vi "create_measure_log_entry.vi"(0 "Messlogbuch-Pfad":path, 1 "Probe":string, 2 "Polarisation [°]":dbl, 3 "Messart":string, 4 "ROI":i32[](array[numeric]), 5 "error in":errorcluster, 6 "Messungen/Messschritt":i32, 7 "Maximalleistung (iK) [mW]":dbl, 8 "Tip-Spannung [V]":dbl, 9 "Suppressor-Spannung [V]":dbl, 10 "Zeit/Messschritt [ms]":i32, 11 "MCP-Spannung [V]":dbl, 12 "Zeit/Messung [ms]":i32, 13 "Phosphorschirm-Spannung [V]":dbl, 15 "xyz [mm]":dbl[](array[numeric])) -> (14 "Messung Nr.":i32, 19 "error out":errorcluster)   [LabVIEW 2009]
panel:
  out "Gestartet":timestamp
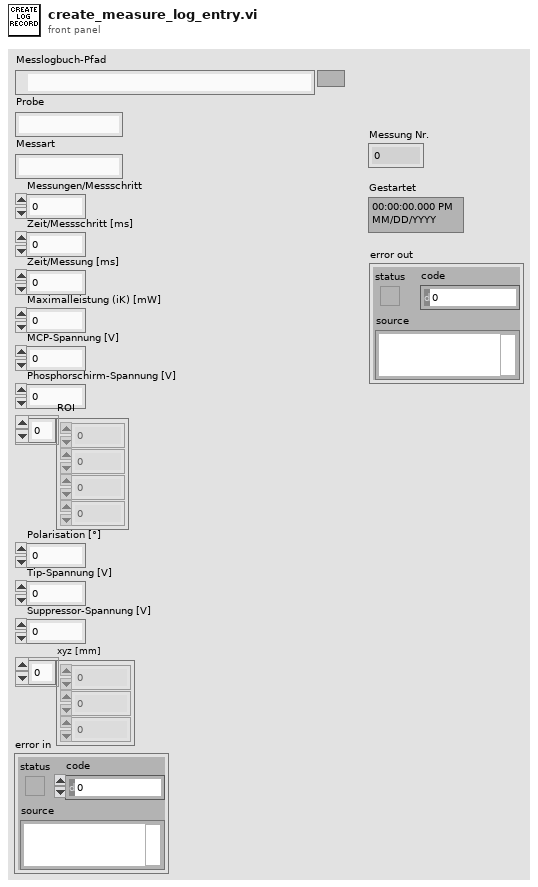
[diagram p1: front panel]
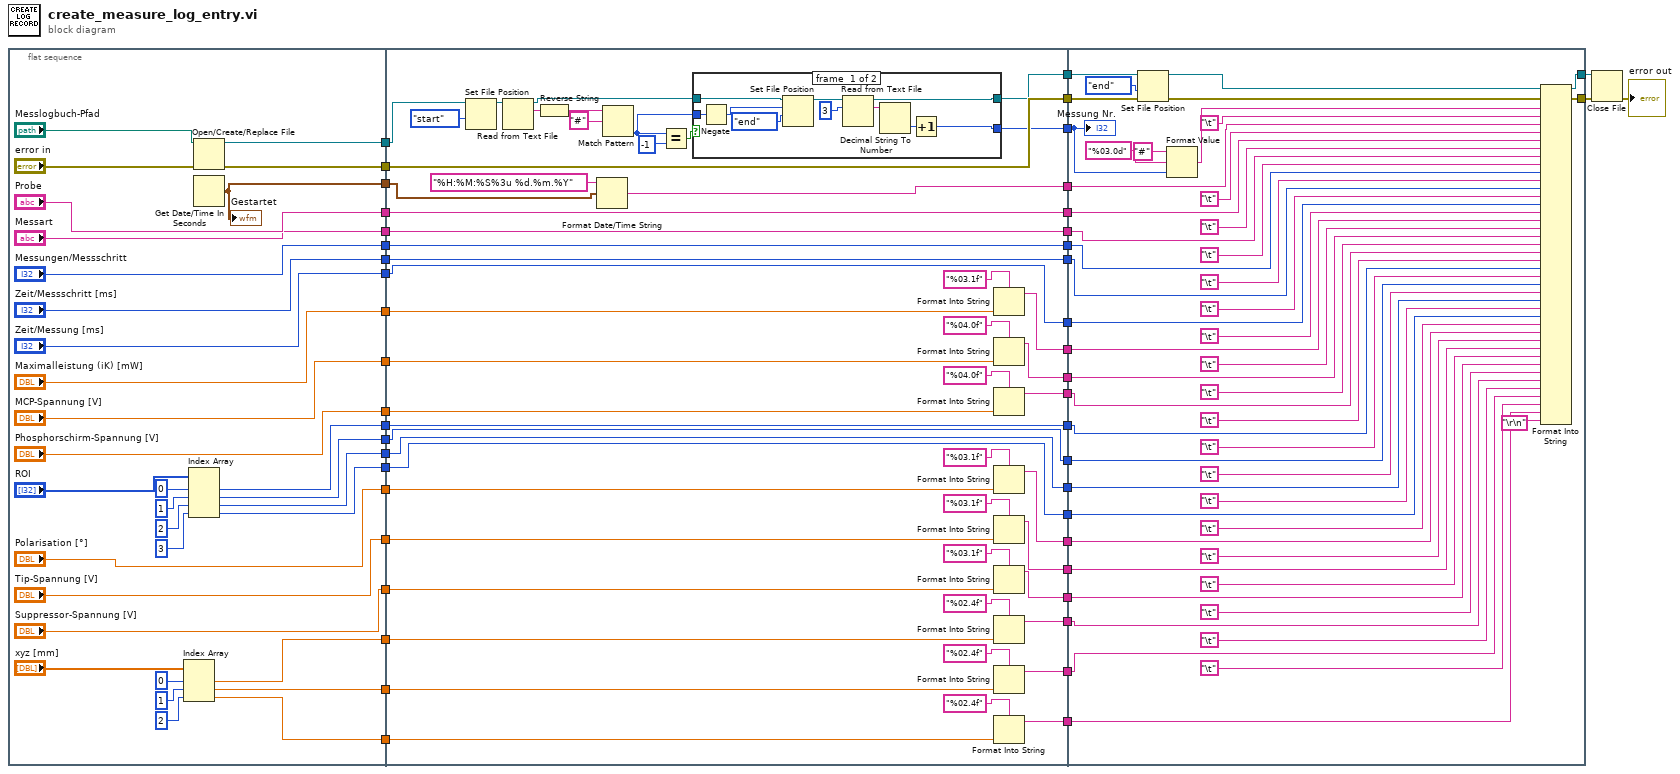
[diagram p0: block diagram]
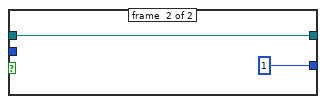
[diagram p2: hidden frame]
diagram:
  n1 = flat-sequence {
    tunnel: ["Probe"] -> w44
    tunnel: ["Messart"] -> w42
    tunnel: ["Messungen/Messschritt"] -> w40
    tunnel: ["Zeit/Messschritt [ms]"] -> w38
    tunnel: ["Zeit/Messung [ms]"] -> w36
    tunnel: ["Maximalleistung (iK) [mW]"] -> w34
    tunnel: ["MCP-Spannung [V]"] -> w32
    tunnel: ["Phosphorschirm-Spannung [V]"] -> w30
    tunnel: [w60] -> w28
    tunnel: [w59] -> w26
    tunnel: [w58] -> w24
    tunnel: [w57] -> w22
    tunnel: [w70] -> w20
    tunnel: [w68] -> w19
    tunnel: [w67] -> w18
    tunnel: ["Polarisation [°]"] -> w12
    tunnel: ["Tip-Spannung [V]"] -> w10
    tunnel: ["Suppressor-Spannung [V]"] -> w8
    tunnel: [w49] -> w6
    tunnel: [w48] -> w4
    tunnel: [w47] -> w2
    tunnel: w44 -> [w130]
    tunnel: [w130] -> w43
    tunnel: w42 -> [w129]
    tunnel: [w129] -> w41
    tunnel: w40 -> [w128]
    tunnel: [w128] -> w39
    tunnel: w38 -> [w127]
    tunnel: [w127] -> w37
    tunnel: w36 -> [w126]
    tunnel: [w126] -> w35
    tunnel: w34 -> [w107]
    tunnel: [w106] -> w33
    tunnel: w32 -> [w101]
    tunnel: [w100] -> w31
    tunnel: w30 -> [w103]
    tunnel: [w102] -> w29
    tunnel: w28 -> [w125]
    tunnel: [w125] -> w27
    tunnel: w26 -> [w124]
    tunnel: [w124] -> w25
    tunnel: w24 -> [w123]
    tunnel: [w123] -> w23
    tunnel: w22 -> [w122]
    tunnel: [w122] -> w21
    tunnel: w20 -> [w80]
    tunnel: w19 -> [w115]
    tunnel: w18 -> [w121]
    tunnel: [w121] -> w17
    tunnel: [w111] -> w16
    tunnel: [w109] -> w15
    tunnel: [w86] -> w13
    tunnel: w12 -> [w87]
    tunnel: [w90] -> w11
    tunnel: w10 -> [w92]
    tunnel: [w89] -> w9
    tunnel: w8 -> [w91]
    tunnel: [w95] -> w7
    tunnel: w6 -> [w98]
    tunnel: [w94] -> w5
    tunnel: w4 -> [w97]
    tunnel: [w93] -> w3
    tunnel: w2 -> [w96]
    tunnel: [w79] -> w1
    tunnel: w43 -> [w179]
    tunnel: w41 -> [w178]
    tunnel: w39 -> [w177]
    tunnel: w37 -> [w176]
    tunnel: w35 -> [w175]
    tunnel: w33 -> [w174]
    tunnel: w31 -> [w173]
    tunnel: w29 -> [w172]
    tunnel: w27 -> [w171]
    tunnel: w25 -> [w170]
    tunnel: w23 -> [w169]
    tunnel: w21 -> [w168]
    tunnel: [w165] -> w46
    tunnel: [w163] -> w45
    tunnel: w17 -> [w162]
    tunnel: w16 -> [w158]
    tunnel: w15 -> [w157]
    tunnel: w13 -> [w150]
    tunnel: w11 -> [w149]
    tunnel: w9 -> [w148]
    tunnel: w7 -> [w147]
    tunnel: w5 -> [w146]
    tunnel: w3 -> [w145]
    tunnel: w1 -> [w143]
    frame #0 {
      n2 = Index Array(array="xyz [mm]", index #1=0 ("index"), index #2=1 ("index"), index #3=2 ("index")) -> (element #1=w49:dbl, element #2=w48:dbl, element #3=w47:dbl)
      n3 = Index Array(array="ROI", index #1=0 ("index"), index #2=1 ("index"), index #3=2 ("index"), index #4=3 ("index")) -> (element #1=w60:i32, element #2=w59:i32, element #3=w58:i32, element #4=w57:i32)
      n4 = Open/Create/Replace File(file path (use dialog)="Messlogbuch-Pfad", error in="error in") -> (refnum out=w68:refnum<file>, error out=w67:errorcluster)  [unwired: 4 in, 1 out]
      n5 = Get Date/Time In Seconds() -> (seconds since 1Jan1904=w70:timestamp)
      "Gestartet" <- w70
    }
    frame #1 {
      n6 = Set File Position(refnum=w115, from (0:start)=enum16{"start", "end", "current"}."start") -> (refnum out=w120:refnum<file>)  [unwired: 2 in, 1 out]
      n7 = Read from Text File(file (use dialog)=w120) -> (refnum out=w110:refnum<file>, text=w117:string)  [unwired: 3 in, 2 out]
      n8 = Reverse String(1:w117) -> (0:w118:string)
      n9 = Format Date/Time String(time format string (%c)="%H:%M:%S%3u %d.%m.%Y" ("Zeitformatierungs-String (%c)"), seconds (now)=w80) -> (date/time string=w79:string)  [unwired: 1 in]
      n10 = Match Pattern(string=w118, regular expression="#" ("search string/char (-)")) -> (offset past match=w112:i32)  [unwired: 1 in, 3 out]
      n11 = Equal?(x=w112, y=-1) -> (x = y?=w113:bool)
      n12 = case shown="False" w113 {
        tunnel: w112 -> [w135 _]
        tunnel: [w133 1] -> w111
        tunnel: w110 -> [w132 w141]
        tunnel: [w131 w141] -> w109
        frame #0 {
          n13 = Negate(x=w135) -> (-x=w137:i32)
          n14 = Set File Position(offset (in bytes) (0)=w137, refnum=w132, from (0:start)=enum16{"start", "end", "current"}."end") -> (refnum out=w138:refnum<file>)  [unwired: 1 in, 1 out]
          n15 = Read from Text File(file (use dialog)=w138, count=3) -> (refnum out=w131:refnum<file>, text=w140:string)  [unwired: 2 in, 2 out]
          n16 = Decimal String To Number(string=w140) -> (number=w134:i32)  [unwired: 2 in, 1 out]
          n17 = Increment(x=w134) -> (x+1=w133:i32)
        }
        frame #1 {
        }
      }
      n18 = Format Into String(format string="%03.1f" ("Format-String"), w107) -> (resulting string=w106:string)  [unwired: 2 in, 1 out]
      n19 = Format Into String(format string="%04.0f" ("Format-String"), w101) -> (resulting string=w100:string)  [unwired: 2 in, 1 out]
      n20 = Format Into String(format string="%04.0f" ("Format-String"), w103) -> (resulting string=w102:string)  [unwired: 2 in, 1 out]
      n21 = Format Into String(format string="%03.1f" ("Format-String"), w87) -> (resulting string=w86:string)  [unwired: 2 in, 1 out]
      n22 = Format Into String(format string="%03.1f" ("Format-String"), w92) -> (resulting string=w90:string)  [unwired: 2 in, 1 out]
      n23 = Format Into String(format string="%03.1f" ("Format-String"), w91) -> (resulting string=w89:string)  [unwired: 2 in, 1 out]
      n24 = Format Into String(format string="%02.4f" ("Format-String"), w98) -> (resulting string=w95:string)  [unwired: 2 in, 1 out]
      n25 = Format Into String(format string="%02.4f" ("Format-String"), w97) -> (resulting string=w94:string)  [unwired: 2 in, 1 out]
      n26 = Format Into String(format string="%02.4f" ("Format-String"), w96) -> (resulting string=w93:string)  [unwired: 2 in, 1 out]
    }
    frame #2 {
      n27 = Set File Position(refnum=w157, from (0:start)=enum16{"start", "end", "current"}."end", error in=w162) -> (refnum out=w166:refnum<file>, error out=w164:errorcluster)  [unwired: 1 in]
      n28 = Format Value(string ("")="#" ("string"), format string="%03.0d", value (0)=w158) -> (output string=w159:string)
      n29 = Format Into String(initial string=w166, error in=w164, w159, "\t", w143, "\t", w179, "\t", w178, "\t", w177, "\t", w176, "\t", w175, "\t", w174, "\t", w173, "\t", w172, "\t", w171, "\t", w170, "\t", w169, "\t", w168, "\t", w150, "\t", w149, "\t", w148, "\t", w147, "\t", w146, "\t", w145, "\r\n") -> (resulting string=w165:refnum<file>, error out=w163:errorcluster)  [unwired: 1 in]
      "Messung Nr." <- w158
    }
  }
  n30 = Close File(refnum=w46, error in=w45) -> (error out=→"error out":errorcluster)  [unwired: 1 out]
